vi "MPVSenden_ECD.vi"(3 "Ventilposition":i32=1 min=1 max=6 step=1, 4 "error in":errorcluster, 5 "FPGA-VI-Referenz":refnum<k20>) -> (0 "Ventilposition":i32, 1 "error out":errorcluster, 2 "FPGA-VI-Referenz (Ausgang)":refnum<k20>)   [LabVIEW 2017]
uses:
  GVVentilposition.vi
  <vilib>/Utility/error.llb/Error Cluster From Error Code.vi
  <vilib>/rvi/errors/niLvFpgaAdjustHostInterfaceError.vi
  <vilib>/rvi/interface/nirviMethod/nirviMethod.xnode
  FPGA Bitfiles/HAGAR-VECD_FPGATarget_FPGA-ProgrammECD_WS++LmW9gGg.lvbitx
  FPGA-Programm_ECD.vi
  <vilib>/FPGAPlugInAG/cRIO-9035/niLvFpga_WriteFifo_cRIO-9035.vi
  <vilib>/rvi/errors/niLvFpgaMergeErrorWithErrorCode.vi
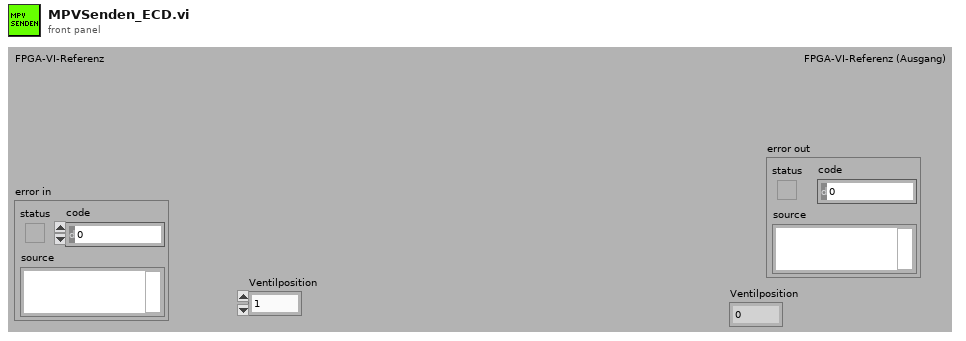
[diagram p1: front panel]
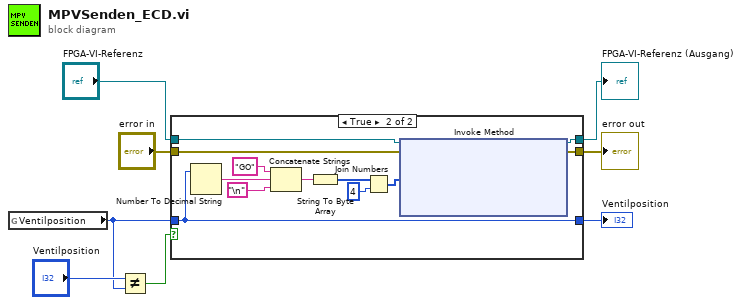
[diagram p0: block diagram]
diagram:
  n1 = global read "GVVentilposition.vi" "Ventilposition"() -> (w6:i32)
  n2 = Not Equal?(x="Ventilposition", y=w6) -> (x != y?=w7:bool)
  n3 = case shown="True" w7 {
    tunnel: "FPGA-VI-Referenz" -> [w11 w23]
    tunnel: [w11 w15] -> w2
    tunnel: w6 -> [w10 w14]
    tunnel: [w10 w14] -> w5
    tunnel: "error in" -> [w9 w13]
    tunnel: [w9 w12] -> w3
    frame False {
    }
    frame True {
      n4 = Number To Decimal String(number=w14) -> (decimal integer string=w16:string)  [unwired: 1 in]
      n5 = Concatenate Strings("GO", w16, "\n") -> (w21:string)
      n6 = String To Byte Array(string=w21) -> (unsigned byte array=w20:u8[])
      n7 = Join Numbers(hi=w20, lo=u8 4) -> ((hi.lo)=w18:u16[])
      n8 = xnode "Invoke Method"("FPGA-VI-Referenz (Eingang)"=w23, "Fehler (Eingang)"=w13, "Daten"=w18) -> ("FPGA-VI-Referenz (Ausgang)"=w15:refnum<k20>, "Fehler (Ausgang)"=w12:errorcluster)  [unwired: 1 in, 1 out]
    }
  }
  "Ventilposition" <- w5
  "error out" <- w3
  "FPGA-VI-Referenz (Ausgang)" <- w2
